vi "GlobalFavorites.vi"() -> ()   [LabVIEW 2013]
panel:
  out "Favorites":bool[](array[boolean])
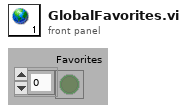
[diagram p1: front panel]
diagram:
